vi "Create FFT Plan 64f.vi"(5 "Direction":T1, 7 "FFT Types":T2, 8 "Error In":errorcluster, 9 "Dimension":T4={"Depth"=1, "Height"=1, "Width"=1} {"Width" min=1; "Height" min=1; "Depth" min=1}, 10 "FFT Dimension":T3, 11 "Labview Device":T5) -> (0 "Error Out":errorcluster, 1 "FFT Output Dimensions":T4={"Depth"=1, "Height"=1, "Width"=1} {"Width" min=1; "Height" min=1; "Depth" min=1}, 3 "FFT Object":T6 {"Imag"."Dimension"."Width" min=1; "Imag"."Dimension"."Height" min=1; "Imag"."Dimension"."Depth" min=1; "Real"."Dimension"."Width" min=1; "Real"."Dimension"."Height" min=1; "Real"."Dimension"."Depth" min=1})   [LabVIEW 2012, in "OpenCLV x64.lvlib"]
doc: "Creates a 64f FFT plan using the input values. This FFT plan stays in memory and can be re-used until destroyed. Any plan created <b>must</b> be destroyed. Allocates a memory buffer that is the proper size based on the type of FFT."
uses:
  OpenCLV x64.lvlib
  FFT Control.ctl
  Controls/Device ID.ctl
  FFT Types.ctl
  FFT Dimension.ctl
  Controls/Memory Object.ctl
  Controls/Memory ID.ctl
  User Controls/Array Dimensions.ctl
  Controls/Memory Type.ctl
  FFT Direction.ctl
  Error Checking/Add Error Functional Global.vi
  Allocate Memory/AllocateMemory_64f.vi
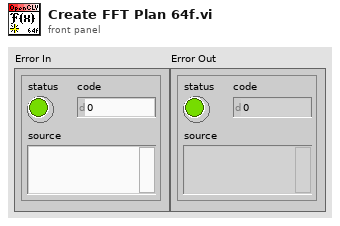
[diagram p1: front panel]
types:
  T1 = typedef "OpenCLV x64.lvlib/FFT Direction.ctl" = enum16{"Forward", "Reverse"}
  T2 = typedef "OpenCLV x64.lvlib/FFT Types.ctl" = enum16{"Real to Hermitian", "Hermitian to Real", "Complex to Complex"}
  T3 = typedef "OpenCLV x64.lvlib/FFT Dimension.ctl" = enum16{"1D FFT", "2D FFT", "3D FFT"}
  T4 = typedef "Array Dimensions.ctl" = cluster{"Depth":u64, "Height":u64, "Width":u64}
  T5 = typedef "OpenCLV x64.lvlib/Device ID.ctl" = u64
  T6 = typedef "OpenCLV x64.lvlib/FFT Control.ctl" = cluster{"Device ID":T5, "FFT Types":T2, "FFT Dim":T3, "Real":T7, "Imag":T7, "FFT Plan":u64, "FFT Direction":T1}
  T7 = typedef "OpenCLV x64.lvlib/Memory Object.ctl" = cluster{"Device ID":T5, "Memeroy ID":T8, "Dimension":T4, "Memory Type":T9}
  T8 = typedef "OpenCLV x64.lvlib/Memory ID.ctl" = u64
  T9 = typedef "OpenCLV x64.lvlib/Memory Type.ctl" = enum16{"32f", "u8", "i8", "u16", "i16", "u32", "i32", "64f"}
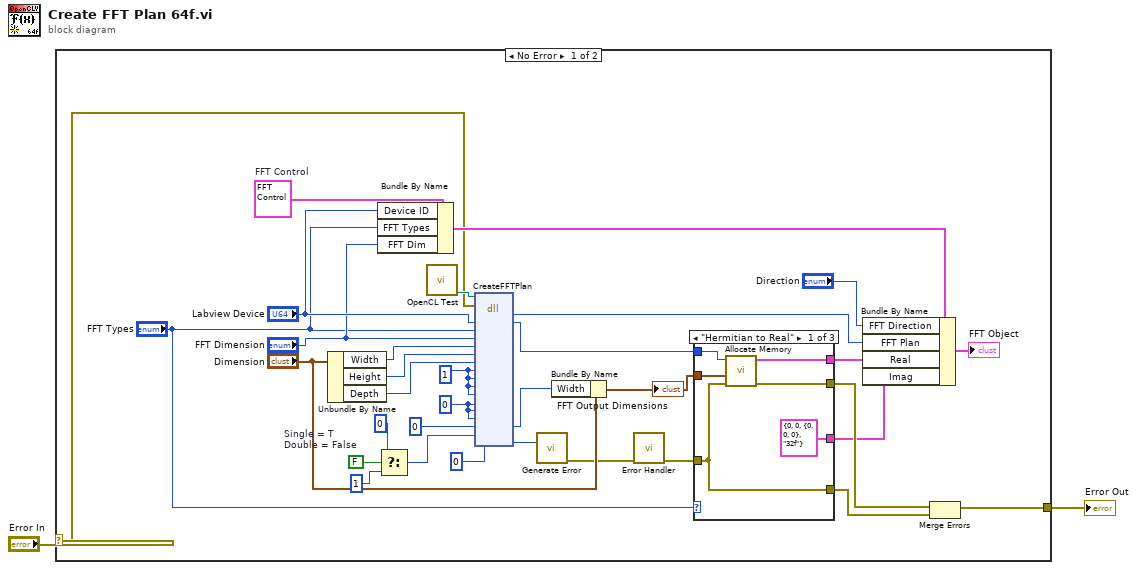
[diagram p0: block diagram]
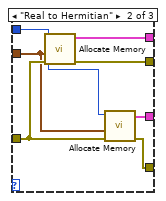
[diagram p2: hidden frame]
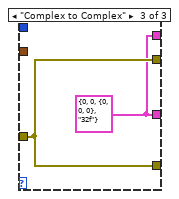
[diagram p3: hidden frame]
diagram:
  n1 = case shown="No Error" "Error In" {
    selector: "Error In" -> [w3 w51]
    tunnel: [w12 w51] -> w1
    frame No Error {
      w18 = T6 {"Device ID"=0, "FFT Types"=enum."Real to Hermitian", "FFT Dim"=enum."1D FFT", "Real"={"Device ID"=0, "Memeroy ID"=0, "Dimension"={"Depth"=0, "Height"=0, "Width"=0}, "Memory Type"=enum."32f"}, "Imag"={"Device ID"=0, "Memeroy ID"=0, "Dimension"={"Depth"=0, "Height"=0, "Width"=0}, "Memory Type"=enum."32f"}, "FFT Plan"=0, "FFT Direction"=enum."Forward"}  # FFT Control
      w33 = FALSE  # Single = T Double = False
      w23 = 0 ("StrideW")
      w22 = 1 ("StrideW")
      n2 = Unbundle By Name("Dimension") -> ("Width"=w19:u64, "Height"=w20:u64, "Depth"=w21:u64)
      n3 = Bundle By Name(cluster=w18, "Device ID"="Labview Device", "FFT Types"="FFT Types", "FFT Dim"="FFT Dimension") -> (w15:T6)
      n4 = Select(t=0, s=w33, f=1 ("t")) -> (s? t:f=w32:i32)
      n5 = call "OpenCL Test.vi"() -> ("DLL To Use"=w6:path)  [unwired: 11 in]
      n6 = dll-call lib="C:/Users/bme-amcelroy-la/Desktop/OpenCLV/trunk/OpenCLV_x64_1.0/OpenCLV_x64.dll" fn="CreateFFTPlan"(path in=w6, error in=w3, "Labview Device"="Labview Device", "FFT Type"="FFT Types", "FFT Dimensions"="FFT Dimension", "Width"=w19, "Height"=w20, "Depth"=w21, "StrideW"=w22, "StrideH"=w22, "StrideD"=w22, "StrideT"=w22, "PaddingW"=w23, "PaddingH"=w23, "PaddingD"=w23, "Output Width"=u64 0 ("BufferSize"), "SingleOrDouble"=w32, "Error"=0) -> ("FFT Plan"=w9:u64, "Labview Device"=w10:u64, "Output Width"=w28:u64, "Error"=w26:i32)  [unwired: 14 in, 2 out]
      n7 = call "Generate Error.vi"("Error"=w26) -> ("error out"=w4:errorcluster)  [unwired: 10 in]
      n8 = Bundle By Name(cluster="Dimension", "Width"=w28) -> (w29:T4)
      "FFT Output Dimensions" <- w29
      n9 = call-poly "Error Handler.vi"("Error In"=w4) -> ("Error Out"=w5:errorcluster)  [unwired: 10 in]
      n10 = case shown="\"Hermitian to Real\"" "FFT Types" {
        tunnel: [w37 w48 w50] -> w31
        tunnel: [w41 w47 w50] -> w30
        tunnel: w5 -> [w37 w46 w50]
        tunnel: w29 -> [w40 w45 _]
        tunnel: [w39 w44 w49] -> w14
        tunnel: [T7 {"Device ID"=0, "Memeroy ID"=0, "Dimension"={"Depth"=0, "Height"=0, "Width"=0}, "Memory Type"=enum."32f"} ("Memory Object") w43 w49] -> w13
        tunnel: w10 -> [w38 w42 _]
        frame "Hermitian to Real" {
          n11 = call-poly "Allocate Memory.vi"("Error In"=w37, "Dimension"=w40, "Device In"=w38) -> ("Error Out"=w41:errorcluster, "Memory Object"=w39:T7)  [unwired: 6 in, 1 out]
        }
        frame "Real to Hermitian" {
          n12 = call-poly "Allocate Memory.vi"("Error In"=w46, "Dimension"=w45, "Device In"=w42) -> ("Error Out"=w47:errorcluster, "Memory Object"=w44:T7)  [unwired: 6 in, 1 out]
          n13 = call-poly "Allocate Memory.vi"("Error In"=w46, "Dimension"=w45, "Device In"=w42) -> ("Error Out"=w48:errorcluster, "Memory Object"=w43:T7)  [unwired: 6 in, 1 out]
        }
        frame "Complex to Complex" {
          w49 = T7 {"Device ID"=0, "Memeroy ID"=0, "Dimension"={"Depth"=0, "Height"=0, "Width"=0}, "Memory Type"=enum."32f"} ("Memory Object")
        }
      }
      n14 = Bundle By Name(cluster=w15, "FFT Direction"="Direction", "FFT Plan"=w9, "Real"=w14, "Imag"=w13) -> (→"FFT Object":T6)
      n15 = Merge Errors(w30, w31) -> (w12:errorcluster)
    }
    frame Error {
    }
  }
  "Error Out" <- w1
